vi "2009-2.vi"() -> ()   [LabVIEW 2010]
panel:
  out "x+y":dbl
  in  "y":dbl
  out "appended array":dbl[](array[numeric])
  in  "Numeric":dbl
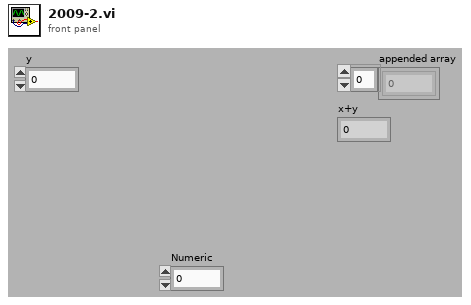
[diagram p1: front panel]
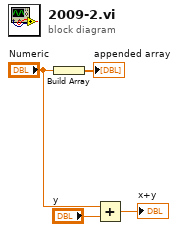
[diagram p0: block diagram]
diagram:
  n1 = Build Array("Numeric") -> (→"appended array":dbl[])
  n2 = Add(x="Numeric", y="y") -> (x+y=→"x+y":dbl)
